vi "Mode selector.vi"(0 "MASTER":i32=1 min=1 max=10 step=1, 1 "IP":string="192.168.23.100", 2 "Mode selector":T1(ring), 5 "PORT":i32=1 min=1 max=4 step=1, 7 "OFF t / ON t":bool, 9 "PWM":i8=50 min=10 max=100 step=1, 11 "error in (no error)":errorcluster, 12 "ON/OFF TIMER (Hour)":i16(knob)=1 min=0 max=24 step=1 scale=0.0..24.0, 13 "ON/OFF TIMER (min)":i16(knob)=1 min=0 max=60 step=1 scale=0.0..60.0, 14 "ON/OFF TIMER (sec)":i16(knob) min=0 max=60 step=1 scale=0.0..60.0) -> (4 "MODE SELECT":string, 6 "Timer in SEC":dbl, 10 "Packet":string, 15 "error out":errorcluster)   [LabVIEW 2022 SP3]
uses:
  <vilib>/NI/Advanced HTTP Client/POST (Buffer).vi
  <vilib>/NI/Advanced HTTP Client/Session.lvclass
panel:
  # "Smart Conn mode selector"
  # "IF MODE \"0\" use switch sub vi for the ON/OFF functions. ."
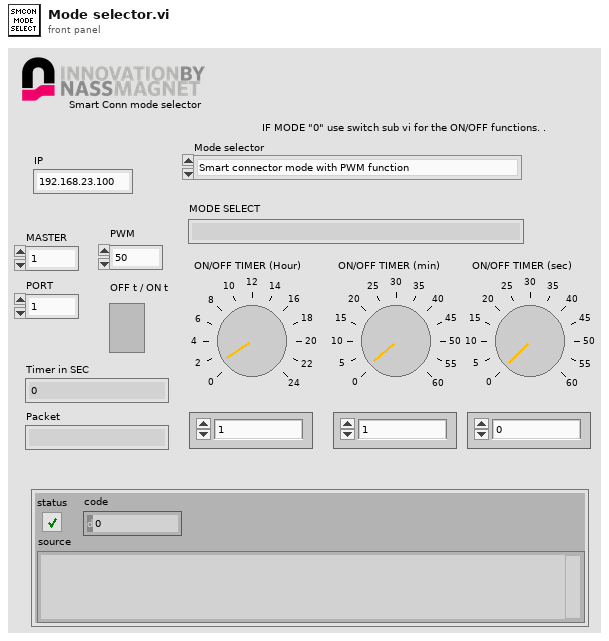
[diagram p1: front panel]
types:
  T1 = enum16{"Smart connector mode with PWM function", "Standard connector mode with PWM function", "On-Off timer with PWM function", "Off - On timer with PWM function", "On delay timer with PWM function (Set Off-time!)", "Off delay timer with PWM function (Set On-time!)"}
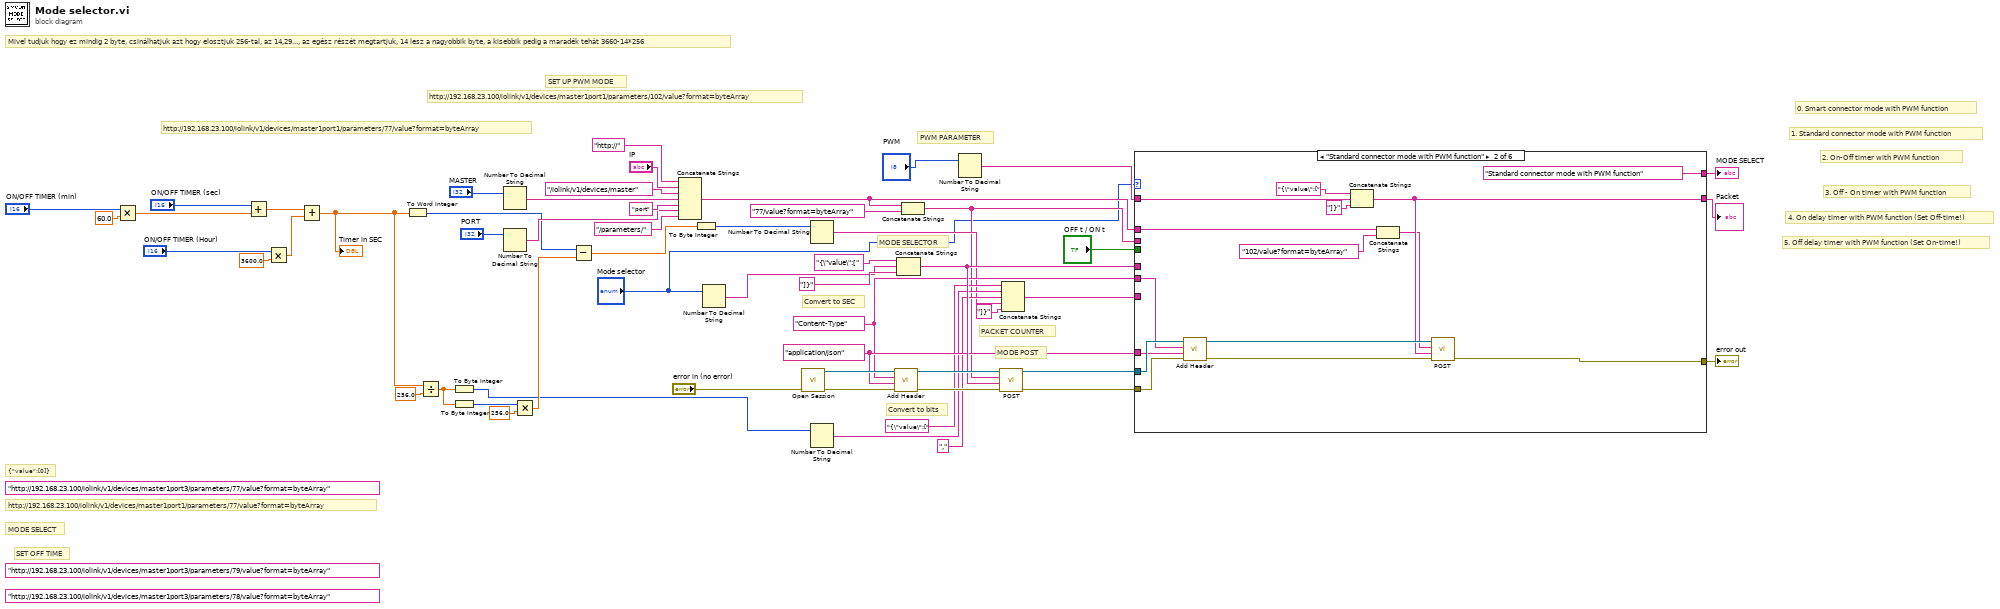
[diagram p0: block diagram]
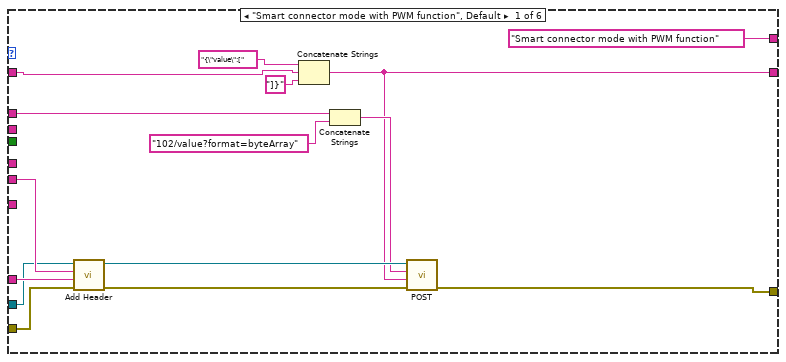
[diagram p2: hidden frame]
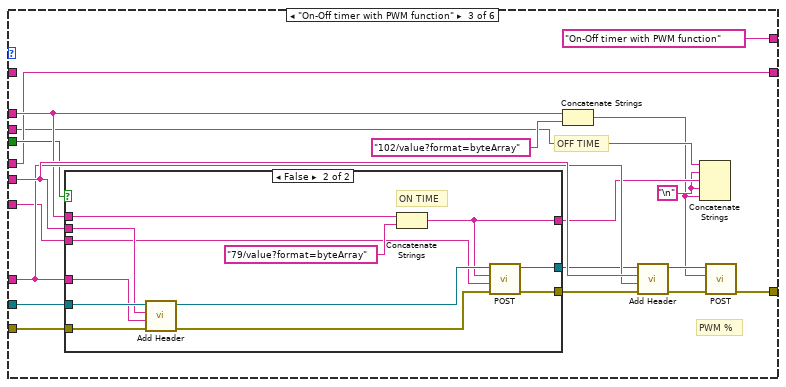
[diagram p3: hidden frame]
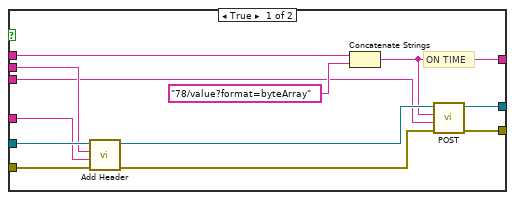
[diagram p4: hidden frame]
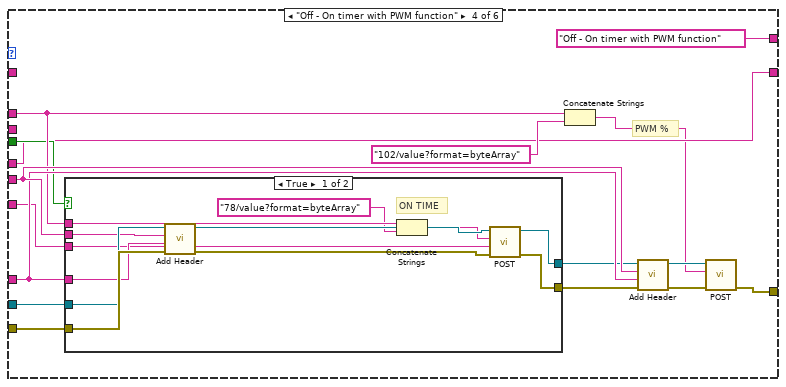
[diagram p5: hidden frame]
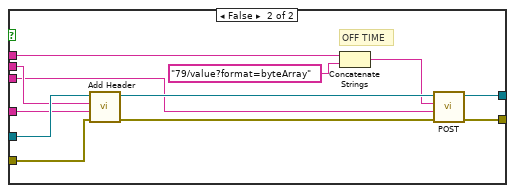
[diagram p6: hidden frame]
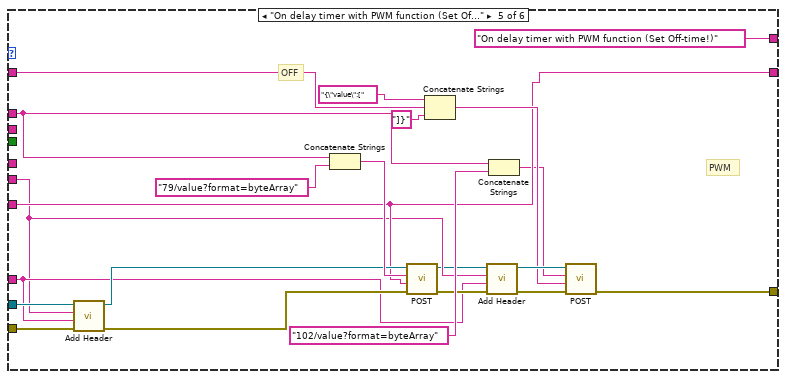
[diagram p7: hidden frame]
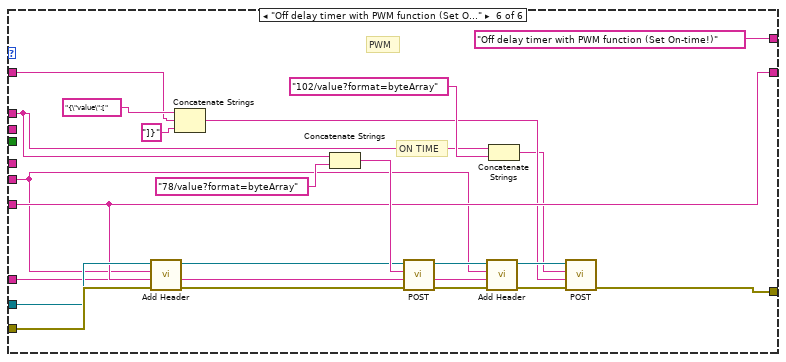
[diagram p8: hidden frame]
diagram:
  (unwired) "http://192.168.23.100/iolink/v1/devices/master1port3/parameters/78/value?format=byteArray" ("url")
  (unwired) "http://192.168.23.100/iolink/v1/devices/master1port3/parameters/79/value?format=byteArray" ("url")
  (unwired) "http://192.168.23.100/iolink/v1/devices/master1port3/parameters/77/value?format=byteArray" ("url")
  w13 = "Content-Type" ("header")
  w14 = "application/json" ("buffer")
  # "5. Off delay timer with PWM function (Set On-time!)"
  # "4. On delay timer with PWM function (Set Off-time!)"
  # "3. Off - On timer with PWM function"
  # "2. On-Off timer with PWM function"
  # "1. Standard connector mode with PWM function"
  # "0. Smart connector mode with PWM function"
  # "PWM PARAMETER"
  # "PACKET COUNTER"
  # "SET UP PWM MODE"
  # "http://192.168.23.100/iolink/v1/devices/master1port1/parameters/102/value?format=byteArray"
  # "MODE POST"
  # "MODE SELECTOR"
  # "Convert to SEC"
  # "Mivel tudjuk hogy ez mindig 2 byte, csinálhatjuk azt hogy elosztjuk 256-tal, az 14,29..., az egész részét megtartjuk, 14 lesz a nagyobbik byte, a kisebbik pedig a maradék tehát 3660-14*256"
  # "Convert to bits"
  # "SET OFF TIME"
  # "MODE SELECT"
  # "http://192.168.23.100/iolink/v1/devices/master1port1/parameters/77/value?format=byteArray"
  # "http://192.168.23.100/iolink/v1/devices/master1port1/parameters/77/value?format=byteArray"
  # "{\"value\":[0]}"
  n1 = Multiply(x="ON/OFF TIMER (min)", y=60.0) -> (x*y=w28:dbl)
  n2 = Add(x="ON/OFF TIMER (sec)", y=w28) -> (x+y=w27:dbl)
  n3 = Multiply(x="ON/OFF TIMER (Hour)", y=3600.0) -> (x*y=w30:dbl)
  n4 = Add(x=w27, y=w30) -> (x+y=w17:dbl)
  "Timer in SEC" <- w17
  n5 = To Word Integer(number=w17) -> (16bit integer=w21:i16)
  n6 = Divide(x=w17, y=256.0) -> (x/y=w23:dbl)
  n7 = To Byte Integer(number=w23) -> (8bit integer=w19:i8)
  n8 = To Byte Integer(number=w23) -> (8bit integer=w24:i8)
  n9 = Number To Decimal String(number="MASTER") -> (decimal integer string=w48:string)  [unwired: 1 in]
  n10 = Number To Decimal String(number="PORT") -> (decimal integer string=w45:string)  [unwired: 1 in]
  n11 = Multiply(x=w24, y=256.0) -> (x*y=w22:dbl)
  n12 = Subtract(x=w21, y=w22) -> (x-y=w20:dbl)
  n13 = Concatenate Strings("http://", "IP", "/iolink/v1/devices/master" ("string"), w48, "port" ("string"), w45, "/parameters/" ("string")) -> (w35:string)
  n14 = To Byte Integer(number=w20) -> (8bit integer=w18:i8)
  n15 = Number To Decimal String(number="Mode selector") -> (decimal integer string=w41:string)  [unwired: 1 in]
  n16 = call <vilib>:"Open Session.vi"("error in"="error in (no error)") -> ("error out"=w53:errorcluster, "session"=w54:refnum<class "Session.lvclass">)  [unwired: 9 in]
  n17 = Number To Decimal String(number=w18) -> (decimal integer string=w6:string)  [unwired: 1 in]
  n18 = Number To Decimal String(number=w19) -> (decimal integer string=w7:string)  [unwired: 1 in]
  n19 = call <vilib>:"Add Header.vi"("error in"=w53, "value"=w14, "header"=w13, "session in"=w54) -> ("error out"=w55:errorcluster, "session out"=w56:refnum<class "Session.lvclass">)  [unwired: 6 in]
  n20 = Concatenate Strings("{\"value\":[" ("buffer"), w41, "]}" ("string")) -> (w15:string)
  n21 = Concatenate Strings(w35, "77/value?format=byteArray" ("string")) -> (w3:string)
  n22 = Number To Decimal String(number="PWM") -> (decimal integer string=w11:string)  [unwired: 1 in]
  n23 = call-poly <vilib>:"POST.vi"("error in"=w55, "buffer"=w15, "url"=w3, "session in"=w56) -> ("error out"=w38:errorcluster, "session out"=w39:refnum<class "Session.lvclass">)  [unwired: 3 in, 3 out]
  n24 = Concatenate Strings("{\"value\":[" ("data"), w7, "," ("string"), w6, "]}" ("string")) -> (w5:string)
  n25 = case shown="\"Standard connector mode with PWM function\"" "Mode selector" {
    tunnel: ["Smart connector mode with PWM function" "Standard connector mode with PWM function" "On-Off timer with PWM function" "Off - On timer with PWM function" "On delay timer with PWM function (Set Off-time!)" "Off delay timer with PWM function (Set On-time!)"] -> w40
    tunnel: w39 -> [w64 w82 w100 w140 w186 w207]
    tunnel: [w70 w85 w104 w144 w171 w199] -> w12
    tunnel: w38 -> [w67 w83 w103 w143 w185 w208]
    tunnel: w35 -> [w61 w79 w93 w133 w172 w196]
    tunnel: [w58 w76 w91 w131 w177 w206] -> w16
    tunnel: w15 -> [_ _ w91 w131 _ _]
    tunnel: w14 -> [w65 w74 w97 w137 w175 w193]
    tunnel: w13 -> [w66 w75 w98 w138 w174 w194]
    tunnel: w11 -> [w57 w73 _ _ w179 w197]
    tunnel: w5 -> [_ _ w96 w136 w177 w206]
    tunnel: "OFF t / ON t" -> [_ _ w92 w132 _ _]
    tunnel: w3 -> [_ _ w90 _ _ _]
    frame "Smart connector mode with PWM function", Default {
      n26 = call <vilib>:"Add Header.vi"("error in"=w67, "value"=w65, "header"=w66, "session in"=w64) -> ("error out"=w68:errorcluster, "session out"=w69:refnum<class "Session.lvclass">)  [unwired: 6 in]
      n27 = Concatenate Strings("{\"value\":[" ("string"), w57, "]}" ("string")) -> (w58:string)
      n28 = Concatenate Strings(w61, "102/value?format=byteArray" ("string")) -> (w63:string)
      n29 = call-poly <vilib>:"POST.vi"("error in"=w68, "buffer"=w58, "url"=w63, "session in"=w69) -> ("error out"=w70:errorcluster)  [unwired: 3 in, 4 out]
    }
    frame "Standard connector mode with PWM function" {
      n30 = call <vilib>:"Add Header.vi"("error in"=w83, "value"=w74, "header"=w75, "session in"=w82) -> ("error out"=w84:errorcluster, "session out"=w81:refnum<class "Session.lvclass">)  [unwired: 6 in]
      n31 = Concatenate Strings("{\"value\":[" ("string"), w73, "]}" ("string")) -> (w76:string)
      n32 = Concatenate Strings(w79, "102/value?format=byteArray" ("string")) -> (w72:string)
      n33 = call-poly <vilib>:"POST.vi"("error in"=w84, "buffer"=w76, "url"=w72, "session in"=w81) -> ("error out"=w85:errorcluster)  [unwired: 3 in, 4 out]
    }
    frame "On-Off timer with PWM function" {
      w88 = "\n"
      # "PWM %"
      # "OFF TIME"
      n34 = case shown="False" w92 {
        tunnel: w103 -> [w116 w128]
        tunnel: w100 -> [w114 w126]
        tunnel: w93 -> [w113 w125]
        tunnel: w98 -> [w111 w123]
        tunnel: w97 -> [w110 w122]
        tunnel: w96 -> [w109 w121]
        tunnel: [w108 w120] -> w95
        tunnel: [w107 w119] -> w94
        tunnel: [w106 w118] -> w89
        frame True {
          # "ON TIME"
          n35 = call <vilib>:"Add Header.vi"("error in"=w116, "value"=w110, "header"=w111, "session in"=w114) -> ("error out"=w117:errorcluster, "session out"=w115:refnum<class "Session.lvclass">)  [unwired: 6 in]
          n36 = Concatenate Strings(w113, "78/value?format=byteArray" ("string")) -> (w106:string)
          n37 = call-poly <vilib>:"POST.vi"("error in"=w117, "buffer"=w109, "url"=w106, "session in"=w115) -> ("error out"=w107:errorcluster, "session out"=w108:refnum<class "Session.lvclass">)  [unwired: 3 in, 3 out]
        }
        frame False {
          # "ON TIME"
          n38 = call <vilib>:"Add Header.vi"("error in"=w128, "value"=w122, "header"=w123, "session in"=w126) -> ("error out"=w129:errorcluster, "session out"=w127:refnum<class "Session.lvclass">)  [unwired: 6 in]
          n39 = Concatenate Strings(w125, "79/value?format=byteArray" ("string")) -> (w118:string)
          n40 = call-poly <vilib>:"POST.vi"("error in"=w129, "buffer"=w121, "url"=w118, "session in"=w127) -> ("error out"=w119:errorcluster, "session out"=w120:refnum<class "Session.lvclass">)  [unwired: 3 in, 3 out]
        }
      }
      n41 = Concatenate Strings(w93, "102/value?format=byteArray" ("string")) -> (w87:string)
      n42 = call <vilib>:"Add Header.vi"("error in"=w94, "value"=w97, "header"=w98, "session in"=w95) -> ("error out"=w102:errorcluster, "session out"=w101:refnum<class "Session.lvclass">)  [unwired: 6 in]
      n43 = Concatenate Strings(w90, w88, w89, w88, w87) -> ()  [unwired: 1 out]
      n44 = call-poly <vilib>:"POST.vi"("error in"=w102, "url"=w87, "session in"=w101) -> ("error out"=w104:errorcluster)  [unwired: 4 in, 4 out]
    }
    frame "Off - On timer with PWM function" {
      # "PWM %"
      n45 = case shown="True" w132 {
        tunnel: w143 -> [w156 w168]
        tunnel: w140 -> [w154 w166]
        tunnel: w133 -> [w153 w165]
        tunnel: w138 -> [w150 w162]
        tunnel: w137 -> [w149 w161]
        tunnel: w136 -> [w148 w160]
        tunnel: [w147 w159] -> w135
        tunnel: [w146 w158] -> w134
        frame True {
          # "ON TIME"
          n46 = call <vilib>:"Add Header.vi"("error in"=w156, "value"=w149, "header"=w150, "session in"=w154) -> ("error out"=w157:errorcluster, "session out"=w155:refnum<class "Session.lvclass">)  [unwired: 6 in]
          n47 = Concatenate Strings(w153, "78/value?format=byteArray" ("string")) -> (w151:string)
          n48 = call-poly <vilib>:"POST.vi"("error in"=w157, "buffer"=w148, "url"=w151, "session in"=w155) -> ("error out"=w146:errorcluster, "session out"=w147:refnum<class "Session.lvclass">)  [unwired: 3 in, 3 out]
        }
        frame False {
          # "OFF TIME"
          n49 = call <vilib>:"Add Header.vi"("error in"=w168, "value"=w161, "header"=w162, "session in"=w166) -> ("error out"=w169:errorcluster, "session out"=w167:refnum<class "Session.lvclass">)  [unwired: 6 in]
          n50 = Concatenate Strings(w165, "79/value?format=byteArray" ("string")) -> (w163:string)
          n51 = call-poly <vilib>:"POST.vi"("error in"=w169, "buffer"=w160, "url"=w163, "session in"=w167) -> ("error out"=w158:errorcluster, "session out"=w159:refnum<class "Session.lvclass">)  [unwired: 3 in, 3 out]
        }
      }
      n52 = Concatenate Strings(w133, "102/value?format=byteArray" ("string")) -> (w130:string)
      n53 = call <vilib>:"Add Header.vi"("error in"=w134, "value"=w137, "header"=w138, "session in"=w135) -> ("error out"=w142:errorcluster, "session out"=w141:refnum<class "Session.lvclass">)  [unwired: 6 in]
      n54 = call-poly <vilib>:"POST.vi"("error in"=w142, "url"=w130, "session in"=w141) -> ("error out"=w144:errorcluster)  [unwired: 4 in, 4 out]
    }
    frame "On delay timer with PWM function (Set Off-time!)" {
      # "OFF"
      # "PWM"
      n55 = call <vilib>:"Add Header.vi"("error in"=w185, "value"=w175, "header"=w174, "session in"=w186) -> ("error out"=w188:errorcluster, "session out"=w187:refnum<class "Session.lvclass">)  [unwired: 6 in]
      n56 = Concatenate Strings(w172, "79/value?format=byteArray" ("string")) -> (w190:string)
      n57 = call-poly <vilib>:"POST.vi"("error in"=w188, "buffer"=w177, "url"=w190, "session in"=w187) -> ("error out"=w176:errorcluster, "session out"=w173:refnum<class "Session.lvclass">)  [unwired: 3 in, 3 out]
      n58 = Concatenate Strings("{\"value\":[" ("string"), w179, "]}" ("string")) -> (w178:string)
      n59 = call <vilib>:"Add Header.vi"("error in"=w176, "value"=w175, "header"=w174, "session in"=w173) -> ("error out"=w183:errorcluster, "session out"=w184:refnum<class "Session.lvclass">)  [unwired: 6 in]
      n60 = Concatenate Strings(w172, "102/value?format=byteArray" ("string")) -> (w170:string)
      n61 = call-poly <vilib>:"POST.vi"("error in"=w183, "buffer"=w178, "url"=w170, "session in"=w184) -> ("error out"=w171:errorcluster)  [unwired: 3 in, 4 out]
    }
    frame "Off delay timer with PWM function (Set On-time!)" {
      # "PWM"
      # "ON TIME"
      n62 = call <vilib>:"Add Header.vi"("error in"=w208, "value"=w193, "header"=w194, "session in"=w207) -> ("error out"=w209:errorcluster, "session out"=w210:refnum<class "Session.lvclass">)  [unwired: 6 in]
      n63 = Concatenate Strings("{\"value\":[" ("string"), w197, "]}" ("string")) -> (w200:string)
      n64 = Concatenate Strings(w196, "78/value?format=byteArray" ("string")) -> (w211:string)
      n65 = call-poly <vilib>:"POST.vi"("error in"=w209, "buffer"=w206, "url"=w211, "session in"=w210) -> ("error out"=w198:errorcluster, "session out"=w195:refnum<class "Session.lvclass">)  [unwired: 3 in, 3 out]
      n66 = call <vilib>:"Add Header.vi"("error in"=w198, "value"=w193, "header"=w194, "session in"=w195) -> ("error out"=w204:errorcluster, "session out"=w205:refnum<class "Session.lvclass">)  [unwired: 6 in]
      n67 = Concatenate Strings(w196, "102/value?format=byteArray" ("string")) -> (w192:string)
      n68 = call-poly <vilib>:"POST.vi"("error in"=w204, "buffer"=w200, "url"=w192, "session in"=w205) -> ("error out"=w199:errorcluster)  [unwired: 3 in, 4 out]
    }
  }
  "error out" <- w12
  "MODE SELECT" <- w40
  "Packet" <- w16
